vi "damn.vi"() -> ()   [LabVIEW 2021]
panel:
  out "XY Graph":cluster{dbl[], dbl[]}(graph)
  out "displacement":dbl[](array[numeric])
  out "Array":dbl[][](array[numeric])
  in  "file path (use dialog)":path
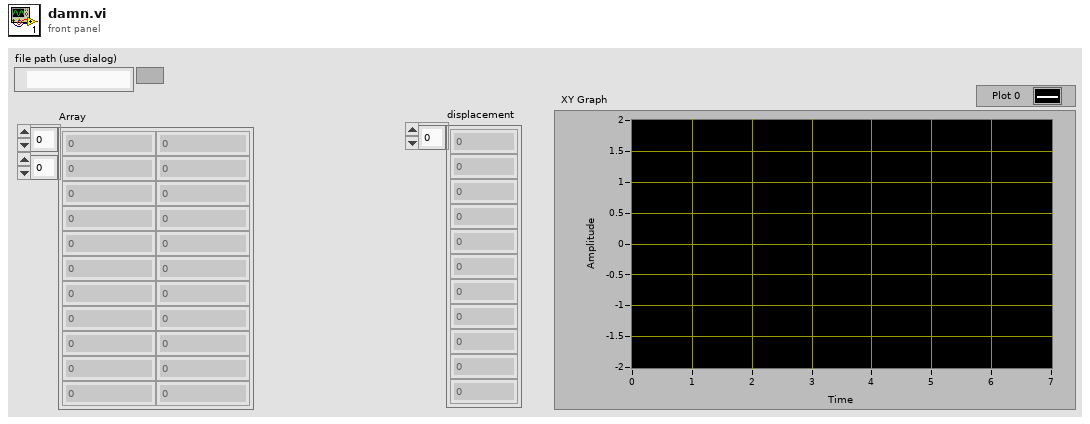
[diagram p1: front panel]
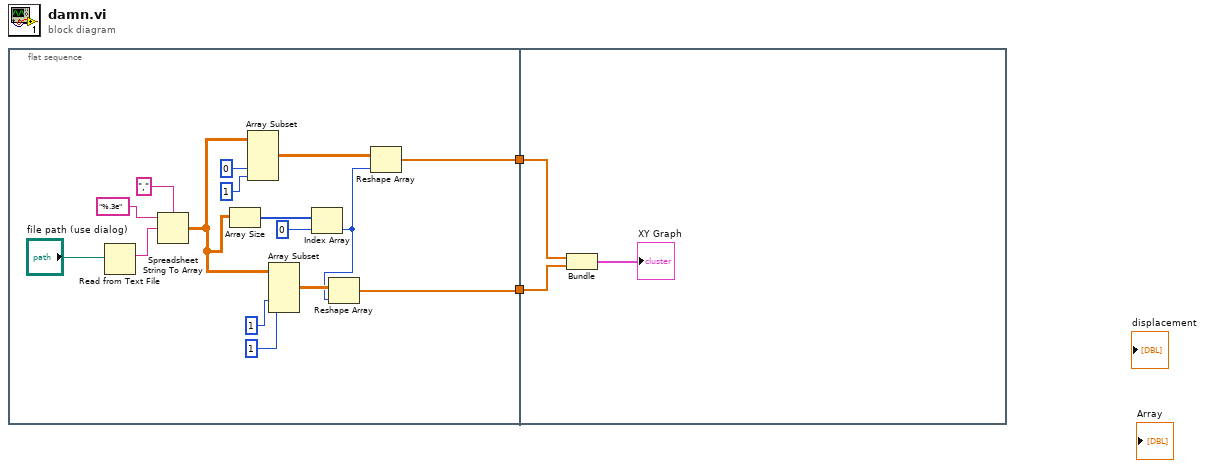
[diagram p0: block diagram]
diagram:
  n1 = flat-sequence {
    tunnel: [w6] -> w2
    tunnel: [w5] -> w1
    tunnel: w2 -> [w19]
    tunnel: w1 -> [w21]
    frame #0 {
      n2 = Read from Text File(file (use dialog)="file path (use dialog)") -> (text=w15:string)  [unwired: 3 in, 3 out]
      n3 = Spreadsheet String To Array(delimiter (Tab)=",", format string="%.3e", spreadsheet string=w15) -> (array=w3:dbl[][])  [unwired: 1 in]
      n4 = Array Size(array=w3) -> (size(s)=w17:i32[])
      n5 = Array Subset(array=w3, index (col)=0 ("index"), length (col)=1 ("length")) -> (w16:dbl[][])  [unwired: 2 in]
      n6 = Array Subset(array=w3, index (col)=1 ("index"), length (col)=1 ("length")) -> (w18:dbl[][])  [unwired: 2 in]
      n7 = Index Array(array=w17, index=0) -> (element=w4:i32)
      n8 = Reshape Array(w18, w4) -> (w5:dbl[])
      n9 = Reshape Array(w16, w4) -> (w6:dbl[])
    }
    frame #1 {
      n10 = Bundle(w19, w21) -> (→"XY Graph":cluster{dbl[], dbl[]})  [unwired: 1 in]
    }
  }
